vi "RequestTrig.vi"(8 "error in (no error)":errorcluster, 10 "Master Device in":refnum<class "Master Device.lvclass">, 11 "ArduinoDAC in":refnum<class "ArduinoDAC.lvclass">) -> (0 "error out":errorcluster, 2 "Master Device out":refnum<class "Master Device.lvclass">, 3 "ArduinoDAC out":refnum<class "ArduinoDAC.lvclass">)   [LabVIEW 2013, in "ArduinoDAC.lvclass"]
doc: "RequestTrig is the second subVI called in PrepareHWI--after ParseSWI.vi. Here, you should compare each ramp (end of last to start of first AND within each ramp) to see whether the device output is changing. For each ramp line, you should build a boolean array (reverse time order!) where TRUE denotes trigger required (i.e. output changes and must be triggered) and FALSE means no trigger is needed. Then pass the boolean array to Update Trigger Line.vi on the Master Device to request triggering.\n\nAfter all devices have a chance to request triggering, in FinalizeHWI.vi, each one will re-check their trigger line and Prune out lines which do not need to be programmed and then BuildHWI."
uses:
  ArduinoDAC.lvclass
  Master Device/Master Device.lvclass
  Device/Device.lvclass
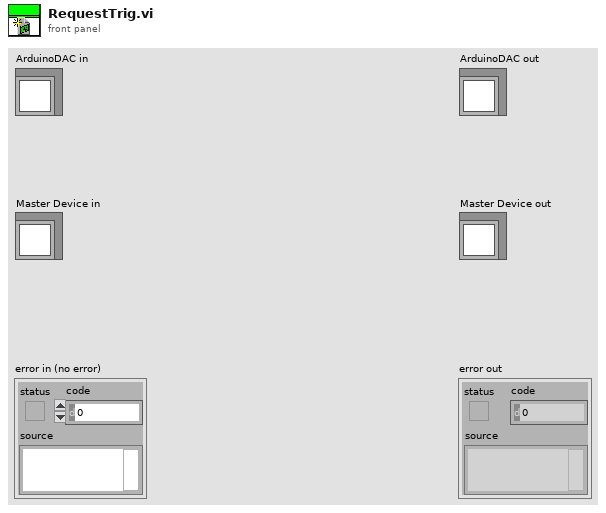
[diagram p1: front panel]
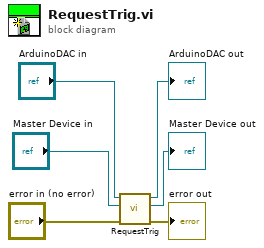
[diagram p0: block diagram]
diagram:
  n1 = call-parent "RequestTrig.vi"("error in (no error)"="error in (no error)", "Master Device in"="Master Device in", "Device in"="ArduinoDAC in") -> ("error out"=→"error out":errorcluster, "Master Device out"=→"Master Device out":refnum<class "Master Device.lvclass">, "Device out"=→"ArduinoDAC out":refnum<class "ArduinoDAC.lvclass">)  [unwired: 6 in]
